vi "StateExecution.vi"(4 "Constant increment":u8, 5 "State out":i16, 6 "Left Grabber":cluster{}, 7 "LeftServo":cluster{"Servo":T1, "Address":i16}, 8 "Right Grabber":cluster{}, 9 "RightServo":cluster{"Servo":T1, "Address":i16}) -> (0 "Left Out":cluster{u8, u8, u8})   [LabVIEW 2010, in "4150_RingItUp_State.lvrbt"]
uses:
  4150_RingItUp_State/4150_RingItUp_State.lvrbt
  <vilib>/NXT/Subs/MotorXNode.Servo Type.ctl
  <vilib>/NXT/Subs/MotorXNode.1Servo.ctl
  <vilib>/NXT/Subs/LVHSConnector.ctl
  <vilib>/NXT/NXTIO Xnodes/NXTIONodeSubVIs/TETRIX IO Move Servos.vi
  <vilib>/NXT/NXTIO Xnodes/NXTIOXNode/NXTIO.xnode
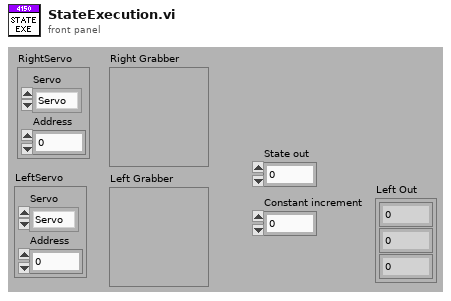
[diagram p1: front panel]
types:
  T1 = typedef "MotorXNode.Servo Type.ctl" = enum16{"Servo"}
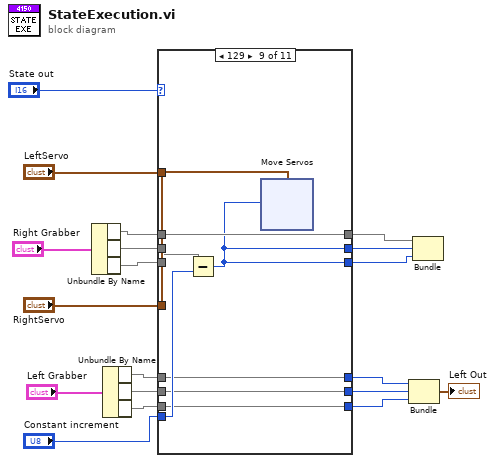
[diagram p0: block diagram]
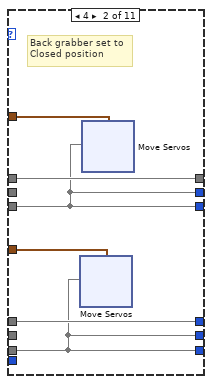
[diagram p3: hidden frame]
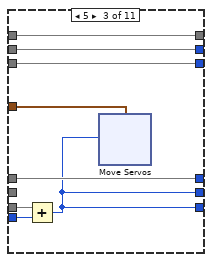
[diagram p4: hidden frame]
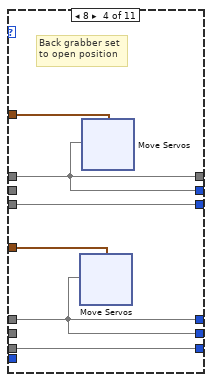
[diagram p5: hidden frame]
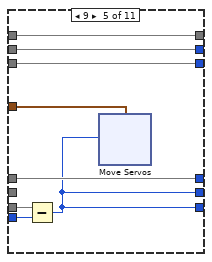
[diagram p6: hidden frame]
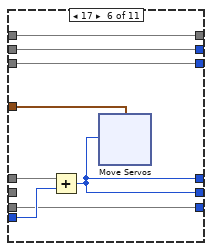
[diagram p7: hidden frame]
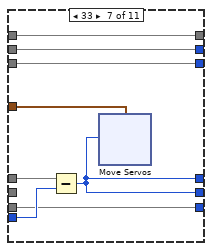
[diagram p8: hidden frame]
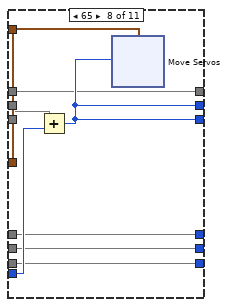
[diagram p9: hidden frame]
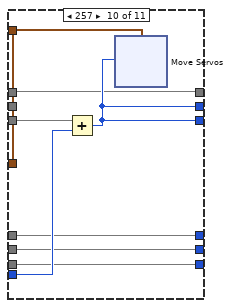
[diagram p10: hidden frame]
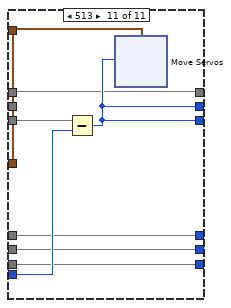
[diagram p11: hidden frame]
diagram:
  n1 = Unbundle By Name("Right Grabber") -> (w8, w7, w6)
  n2 = Unbundle By Name("Left Grabber") -> (w5, w4, w3)
  n3 = case shown="129" "State out" {
    tunnel: "LeftServo" -> [_ w31 _ w69 _ _ _ _ _ _ _]
    tunnel: "RightServo" -> [_ w30 w55 w68 w93 w105 w121 w141 w157 w172 w188]
    tunnel: w6 -> [w23 w28 w48 w67 w86 w106 w122 w139 w155 w171 w187]
    tunnel: w3 -> [w20 w26 w53 w66 w91 w104 w120 w136 w151 w166 w182]
    tunnel: [w24 w28 w49 w65 w87 w107 w123 w138 w153 w170 w186] -> w15
    tunnel: [w23 w28 w48 w67 w86 w106 w122 w138 w153 w170 w186] -> w14
    tunnel: [w25 w29 w50 w65 w88 w108 w124 w137 w154 w169 w185] -> w10
    tunnel: w8 -> [w25 w29 w50 w65 w88 w108 w124 w137 w154 w169 w185]
    tunnel: w5 -> [w22 w27 w54 w64 w92 w103 w119 w134 w150 w168 w184]
    tunnel: w4 -> [w21 _ _ _ _ _ _ w135 w152 w167 w183]
    tunnel: [w22 w27 w54 w64 w92 w102 w118 w134 w150 w168 w184] -> w13
    tunnel: [w20 w26 w51 w66 w89 w104 w120 w136 w151 w166 w182] -> w11
    tunnel: [w21 w26 w51 w64 w89 w102 w118 w135 w152 w167 w183] -> w12
    tunnel: w7 -> [w24 _ w49 _ w87 w107 w123 _ _ _ _]
    tunnel: "Constant increment" -> [_ _ w52 _ w90 w109 w125 w140 w156 w173 w189]
    frame 0, Default {
    }
    frame 4 {
      # "Back grabber set to\nClosed position"
      n4 = xnode ("Move Servos")("Position 1"=w26, "Servos"=w30) -> ()  [unwired: 1 in, 1 out]
      n5 = xnode ("Move Servos")("Position 1"=w28, "Servos"=w31) -> ()  [unwired: 1 in, 1 out]
    }
    frame 5 {
      n6 = Add(x=w53, y=w52) -> (x+y=w51:u8)
      n7 = xnode ("Move Servos")("Position 1"=w51, "Servos"=w55) -> ()  [unwired: 1 in, 1 out]
    }
    frame 8 {
      # "Back grabber set\nto open position"
      n8 = xnode ("Move Servos")("Position 1"=w64, "Servos"=w68) -> ()  [unwired: 1 in, 1 out]
      n9 = xnode ("Move Servos")("Position 1"=w65, "Servos"=w69) -> ()  [unwired: 1 in, 1 out]
    }
    frame 9 {
      n10 = Subtract(x=w91, y=w90) -> (x-y=w89:u8)
      n11 = xnode ("Move Servos")("Position 1"=w89, "Servos"=w93) -> ()  [unwired: 1 in, 1 out]
    }
    frame 17 {
      n12 = Add(x=w103, y=w109) -> (x+y=w102:u8)
      n13 = xnode ("Move Servos")("Position 1"=w102, "Servos"=w105) -> ()  [unwired: 1 in, 1 out]
    }
    frame 33 {
      n14 = Subtract(x=w119, y=w125) -> (x-y=w118:u8)
      n15 = xnode ("Move Servos")("Position 1"=w118, "Servos"=w121) -> ()  [unwired: 1 in, 1 out]
    }
    frame 65 {
      n16 = Add(x=w139, y=w140) -> (x+y=w138:u8)
      n17 = xnode ("Move Servos")("Position 1"=w138, "Servos"=w141) -> ()  [unwired: 1 in, 1 out]
    }
    frame 129 {
      n18 = Subtract(x=w155, y=w156) -> (x-y=w153:u8)
      n19 = xnode ("Move Servos")("Position 1"=w153, "Servos"=w157) -> ()  [unwired: 1 in, 1 out]
    }
    frame 257 {
      n20 = Add(x=w171, y=w173) -> (x+y=w170:u8)
      n21 = xnode ("Move Servos")("Position 1"=w170, "Servos"=w172) -> ()  [unwired: 1 in, 1 out]
    }
    frame 513 {
      n22 = Subtract(x=w187, y=w189) -> (x-y=w186:u8)
      n23 = xnode ("Move Servos")("Position 1"=w186, "Servos"=w188) -> ()  [unwired: 1 in, 1 out]
    }
  }
  n24 = Bundle(w13, w12, w11) -> (→"Left Out":cluster{u8, u8, u8})  [unwired: 1 in]
  n25 = Bundle(w10, w15, w14) -> ()  [unwired: 1 in, 1 out]
